vi "MaxEye_ATE_Save_Configuration_Cluster & Array Header.vi"(10 "Label Name":string, 11 "Class Name":string) -> (2 "End":string, 3 "Begin":string)   [LabVIEW 2021]
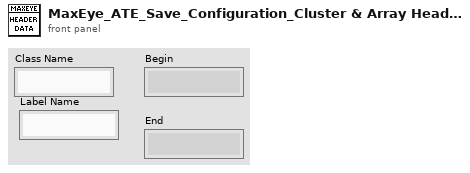
[diagram p1: front panel]
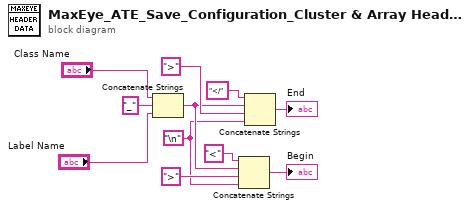
[diagram p0: block diagram]
diagram:
  w1 = "\n"
  n1 = Concatenate Strings("Class Name", "_" ("string"), "Label Name") -> (w2:string)
  n2 = Concatenate Strings("<" ("string"), w2, ">" ("string"), w1) -> (→"Begin":string)
  n3 = Concatenate Strings("</" ("string"), w2, ">" ("string"), w1) -> (→"End":string)
